vi "convertData.vi"(8 "error in (no error)":errorcluster, 10 "continuous":bool=TRUE, 11 "SpinCore in":refnum<class "SpinCore.lvclass">) -> (0 "error out":errorcluster, 2 "Instructions":T1(array[cluster]) {"Op Code" items=["Continue", "Stop", "Loop", "End Loop", "JSR", "RTS", "Branch", "Long Delay", "Wait"]; "Amp Register2" items=["0", "1", "2", "3"]; "Phase Register2" items=["0", "1", "2", "3", "4", "5", "6", "7", "8", "9", "10", "11", "12", "13", "14", "15"]; "Freq Register2" items=["0", "1", "2", "3", "4", "5", "6", "7", "8", "9", "10", "11", "12", "13", "14", "15"]; "Amp Register1" items=["0", "1", "2", "3"]; "Phase Register1" items=["0", "1", "2", "3", "4", "5", "6", "7", "8", "9", "10", "11", "12", "13", "14", "15"]; "Freq Register1" items=["0", "1", "2", "3", "4", "5", "6", "7", "8", "9", "10", "11", "12", "13", "14", "15"]; "Length" format="%.3p"}, 3 "SpinCore out":refnum<class "SpinCore.lvclass">)   [LabVIEW 2011, in "Hardware.lvlib" / "Channels.lvlib" / "SpinCore.lvclass"]
uses:
  SpinCore.lvclass
  SpinCore.lvclass/SpinCore.ctl
panel:
  out "dataChannel0":dbl[][](array[numeric])
  # "0"
  # "1"
  # "2"
  # "3"
  # "4"
  # "5"
  # "6"
  # "7"
  # "8"
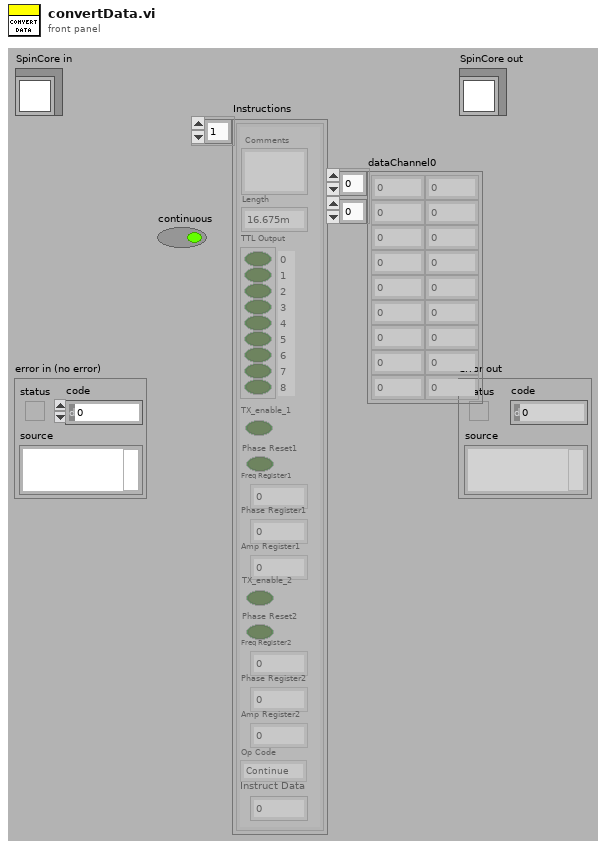
[diagram p1: front panel]
types:
  T1 = cluster{"Comments":string, "Length":dbl, "TTL Output":bool[], "TX_enable_1":bool, "Phase Reset1":bool, "Freq Register1":i32, "Phase Register1":i32, "Amp Register1":i32, "TX_enable_2":bool, "Phase Reset2":bool, "Freq Register2":i32, "Phase Register2":i32, "Amp Register2":i32, "Instruct Data":i32, "Op Code":i32}[]
  T2 = cluster{"Comments":string, "Length":dbl, "TTL Output":bool[], "TX_enable_0":bool, "Phase Reset0":bool, "Freq Register0":i32, "Phase Register0":i32, "Amp Register0":i32, "TX_enable_1":bool, "Phase Reset1":bool, "Freq Register1":i32, "Phase Register1":i32, "Amp Register1":i32, "Instruct Data":i32, "Op Code":i32}[]
  T3 = cluster{"Comments":string, "Length":dbl, "TTL Output":bool[], "TX_enable_1":bool, "Phase Reset1":bool, "Freq Register1":i32, "Phase Register1":i32, "Amp Register1":i32, "TX_enable_2":bool, "Phase Reset2":bool, "Freq Register2":i32, "Phase Register2":i32, "Amp Register2":i32, "Instruct Data":i32, "Op Code":i32}
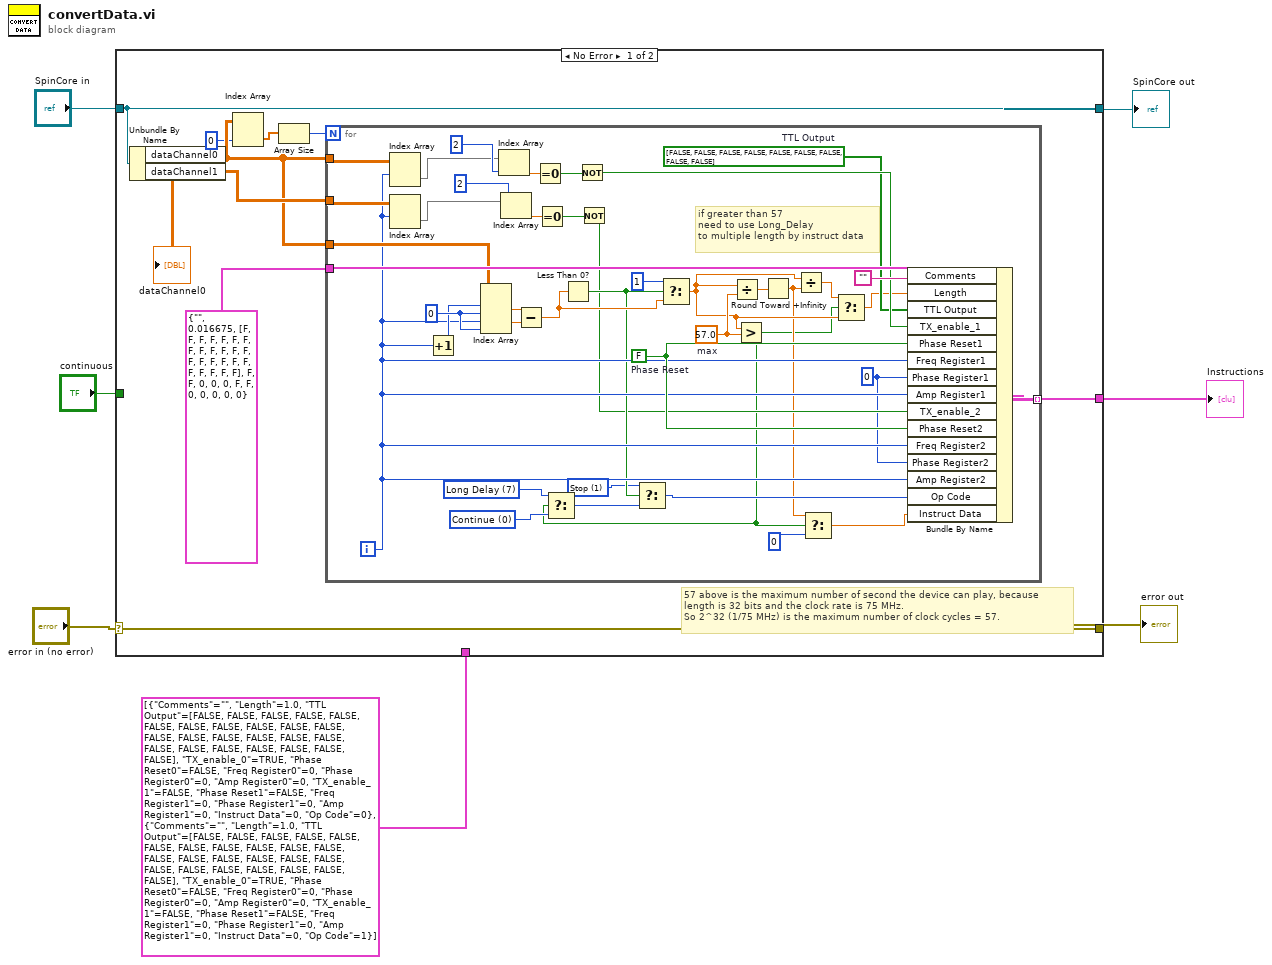
[diagram p0: block diagram]
diagram:
  n1 = case shown="No Error" "error in (no error)" {
    selector: "error in (no error)" -> [w16 w59]
    tunnel: [w16 w59] -> w6
    tunnel: [w15 w58] -> w4
    tunnel: "SpinCore in" -> [w15 w58]
    tunnel: [w8 _] -> w3
    tunnel: T2 [{"Comments"="", "Length"=1.0, "TTL Output"=[FALSE, FALSE, FALSE, FALSE, FALSE, FALSE, FALSE, FALSE, FALSE, FALSE, FALSE, FALSE, FALSE, FALSE, FALSE, FALSE, FALSE, FALSE, FALSE, FALSE, FALSE, FALSE, FALSE, FALSE], "TX_enable_0"=TRUE, "Phase Reset0"=FALSE, "Freq Register0"=0, "Phase Register0"=0, "Amp Register0"=0, "TX_enable_1"=FALSE, "Phase Reset1"=FALSE, "Freq Register1"=0, "Phase Register1"=0, "Amp Register1"=0, "Instruct Data"=0, "Op Code"=0}, {"Comments"="", "Length"=1.0, "TTL Output"=[FALSE, FALSE, FALSE, FALSE, FALSE, FALSE, FALSE, FALSE, FALSE, FALSE, FALSE, FALSE, FALSE, FALSE, FALSE, FALSE, FALSE, FALSE, FALSE, FALSE, FALSE, FALSE, FALSE, FALSE], "TX_enable_0"=TRUE, "Phase Reset0"=FALSE, "Freq Register0"=0, "Phase Register0"=0, "Amp Register0"=0, "TX_enable_1"=FALSE, "Phase Reset1"=FALSE, "Freq Register1"=0, "Phase Register1"=0, "Amp Register1"=0, "Instruct Data"=0, "Op Code"=1}] ("Instructions") -> [_ _]
    tunnel: "continuous" -> [_ _]
    frame No Error {
      # "57 above is the maximum number of second the device can play, because\nlength is 32 bits and the clock rate is 75 MHz.\nSo 2^32 (1/75 MHz) is the maximum number of clock cycles = 57."
      n2 = Unbundle By Name(w15) -> ("dataChannel0"=w13:dbl[][], "dataChannel1"=w14:dbl[][])
      "dataChannel0" <- w13
      n3 = Index Array(array=w13, index (col)=0) -> (element=w12:dbl[])  [unwired: 1 in]
      n4 = Array Size(array=w12) -> (size(s)=w10:i32)
      n5 = for {
        N: w10 -> [_]
        tunnel: w13 -> [w40]
        tunnel: w14 -> [w38]
        tunnel: T3 {"Comments"="", "Length"=0.016675, "TTL Output"=[FALSE, FALSE, FALSE, FALSE, FALSE, FALSE, FALSE, FALSE, FALSE, FALSE, FALSE, FALSE, FALSE, FALSE, FALSE, FALSE, FALSE, FALSE, FALSE, FALSE, FALSE, FALSE, FALSE, FALSE], "TX_enable_1"=FALSE, "Phase Reset1"=FALSE, "Freq Register1"=0, "Phase Register1"=0, "Amp Register1"=0, "TX_enable_2"=FALSE, "Phase Reset2"=FALSE, "Freq Register2"=0, "Phase Register2"=0, "Amp Register2"=0, "Instruct Data"=0, "Op Code"=0} ("DDS-II Instruction") -> [w51]
        tunnel: w13 -> [w49]
        tunnel: [w44] -> w8 mode=indexing
        i -> [w37]
        w17 = 0
        w24 = 57.0  # max
        w28 = 0 items=["Continue", "Stop", "Loop", "End Loop", "JSR", "RTS", "Branch", "Long Delay", "Wait"] ("Op Code")
        w34 = 1 items=["Continue", "Stop", "Loop", "End Loop", "JSR", "RTS", "Branch", "Long Delay", "Wait"] ("Op Code")
        w48 = 0
        w30 = bool[] [FALSE, FALSE, FALSE, FALSE, FALSE, FALSE, FALSE, FALSE, FALSE]  # TTL Output
        w50 = FALSE  # Phase Reset
        w27 = 7 items=["Continue", "Stop", "Loop", "End Loop", "JSR", "RTS", "Branch", "Long Delay", "Wait"] ("Op Code")
        # "if greater than 57\nneed to use Long_Delay\nto multiple length by instruct data"
        n6 = Index Array(array=w40, index (row)=w37) -> (element=w39:dbl[])  [unwired: 1 in]
        n7 = Index Array(array=w38, index (row)=w37) -> (element=w36:dbl[])  [unwired: 1 in]
        n8 = Increment(x=w37) -> (x+1=w47:i32)
        n9 = Index Array(array=w49, index (row) #1=w47, index (col) #1=w48, index (row) #2=w37, index (col) #2=w48) -> (element #1=w46:dbl, element #2=w45:dbl)
        n10 = Index Array(array=w39, index=2) -> (element=w56:dbl)
        n11 = Index Array(array=w36, index=2) -> (element=w53:dbl)
        n12 = Subtract(x=w46, y=w45) -> (x-y=w42:dbl)
        n13 = Equal To 0?(x=w56) -> (x = 0?=w55:bool)
        n14 = Equal To 0?(x=w53) -> (x = 0?=w52:bool)
        n15 = Less Than 0?(x=w42) -> (x < 0?=w35:bool)
        n16 = Not(x=w55) -> (.not. x?=w31:bool)
        n17 = Not(x=w52) -> (.not. x?=w32:bool)
        n18 = Select(t=1, s=w35, f=w42) -> (s? t:f=w21:dbl)
        n19 = Divide(x=w21, y=w24) -> (x/y=w23:dbl)
        n20 = Greater?(x=w21, y=w24) -> (0:w18:bool)
        n21 = Select(t=w27, s=w18, f=w28) -> (s? t:f=w29:i32)
        n22 = Select(t=w34, s=w35, f=w29) -> (s? t:f=w33:i32)
        n23 = Round Toward +Infinity(x=w23) -> (ceil(x): smallest int >= x=w19:dbl)
        n24 = Divide(x=w21, y=w19) -> (x/y=w22:dbl)
        n25 = Select(t=w19, s=w18, f=0) -> (s? t:f=w25:dbl)
        n26 = Select(t=w22, s=w18, f=w21) -> (s? t:f=w20:dbl)
        n27 = Bundle By Name(cluster=w51, "Comments"="", "Length"=w20, "TTL Output"=w30, "TX_enable_1"=w31, "Phase Reset1"=w50, "Freq Register1"=w37, "Phase Register1"=w17, "Amp Register1"=w37, "TX_enable_2"=w32, "Phase Reset2"=w50, "Freq Register2"=w37, "Phase Register2"=w17, "Amp Register2"=w37, "Op Code"=w33, "Instruct Data"=w25) -> (w44:T3)
      }
    }
    frame Error {
    }
  }
  "error out" <- w6
  "SpinCore out" <- w4
  "Instructions" <- w3
